vi "test photon averaging.vi"() -> ()   [LabVIEW 2010]
uses:
  <vilib>/rvi/FXPMathLib/FxpInterpret/XNode/nifxpmath_Interpret.xnode
  <vilib>/rvi/FXPMathLib/FxpSub/XNode/nifxpmath_Sub.xnode
  <vilib>/rvi/FXPMathLib/FxpSub/subVIs/nifxpmath_Sub_SimConfig.ctl
  <vilib>/fxp/LVFixedPointQuantizationPolicyTypeDef.ctl
  <vilib>/fxp/LVFixedPointOverflowPolicyTypeDef.ctl
  <vilib>/rvi/FXPMathLib/FxpAdd/XNode/nifxpmath_Add.xnode
  <vilib>/rvi/FXPMathLib/FxpAdd/subVIs/nifxpmath_Add_SimConfig.ctl
  <vilib>/rvi/FXPMathLib/FxpSub/simVIs/DllFxpSubTemp_sub.vi
  <vilib>/rvi/FXPMathLib/FxpAdd/simVIs/DllFxpAddTemp_sub.vi
panel:
  out "new photon count":fxp<+,32,8> format="%.27g"
  in  "new photons":u32
  in  "old photon count":fxp<+,32,8> format="%.27g"
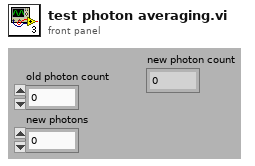
[diagram p1: front panel]
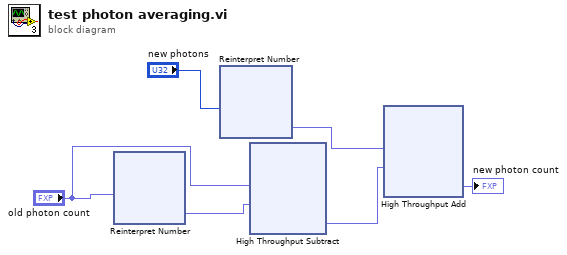
[diagram p0: block diagram]
diagram:
  n1 = xnode "Reinterpret Number"("x"="old photon count") -> ("y"=w6:fxp<+,32,-8>)
  n2 = xnode "Reinterpret Number"("x"="new photons") -> ("y"=w5:fxp<+,32,16>)
  n3 = xnode "High Throughput Subtract"("x"="old photon count", "y"=w6) -> ("x-y"=w4:fxp<+,32,8>)
  n4 = xnode "High Throughput Add"("x"=w5, "y"=w4) -> ("x+y"=→"new photon count":fxp<+,32,8>)
